vi "Init images and labels.vi"(8 "error in (no error)":errorcluster, 9 "JSON Read":T1, 10 "References":T3, 11 "ControlsIndicators":T5) -> (0 "error out":errorcluster)   [LabVIEW 2019, in "ZenGage v3.0 UI.lvclass"]
uses:
  ZenGage v3.0 UI.lvclass
  Type Definitions/Controls and Indicators/Controls and Indicators Cluster.ctl
  Type Definitions/Controls and Indicators/EDL control references.ctl
  Type Definitions/Controls and Indicators/Select a part (combobox).ctl
  Type Definitions/Controls and Indicators/Diagnostics control referencs.ctl
  Type Definitions/Controls and Indicators/Inspection control references.ctl
  Type Definitions/Controls and Indicators/General_Control references.ctl
  Type Definitions/JSON Read/UI JSON read cluster.ctl
  Type Definitions/General/JSONRead.ctl
  Type Definitions/General/Master sample references.ctl
panel:
  out "TL":string
  out "Trigger Diagnostics (TL)":T4(plugin-control)
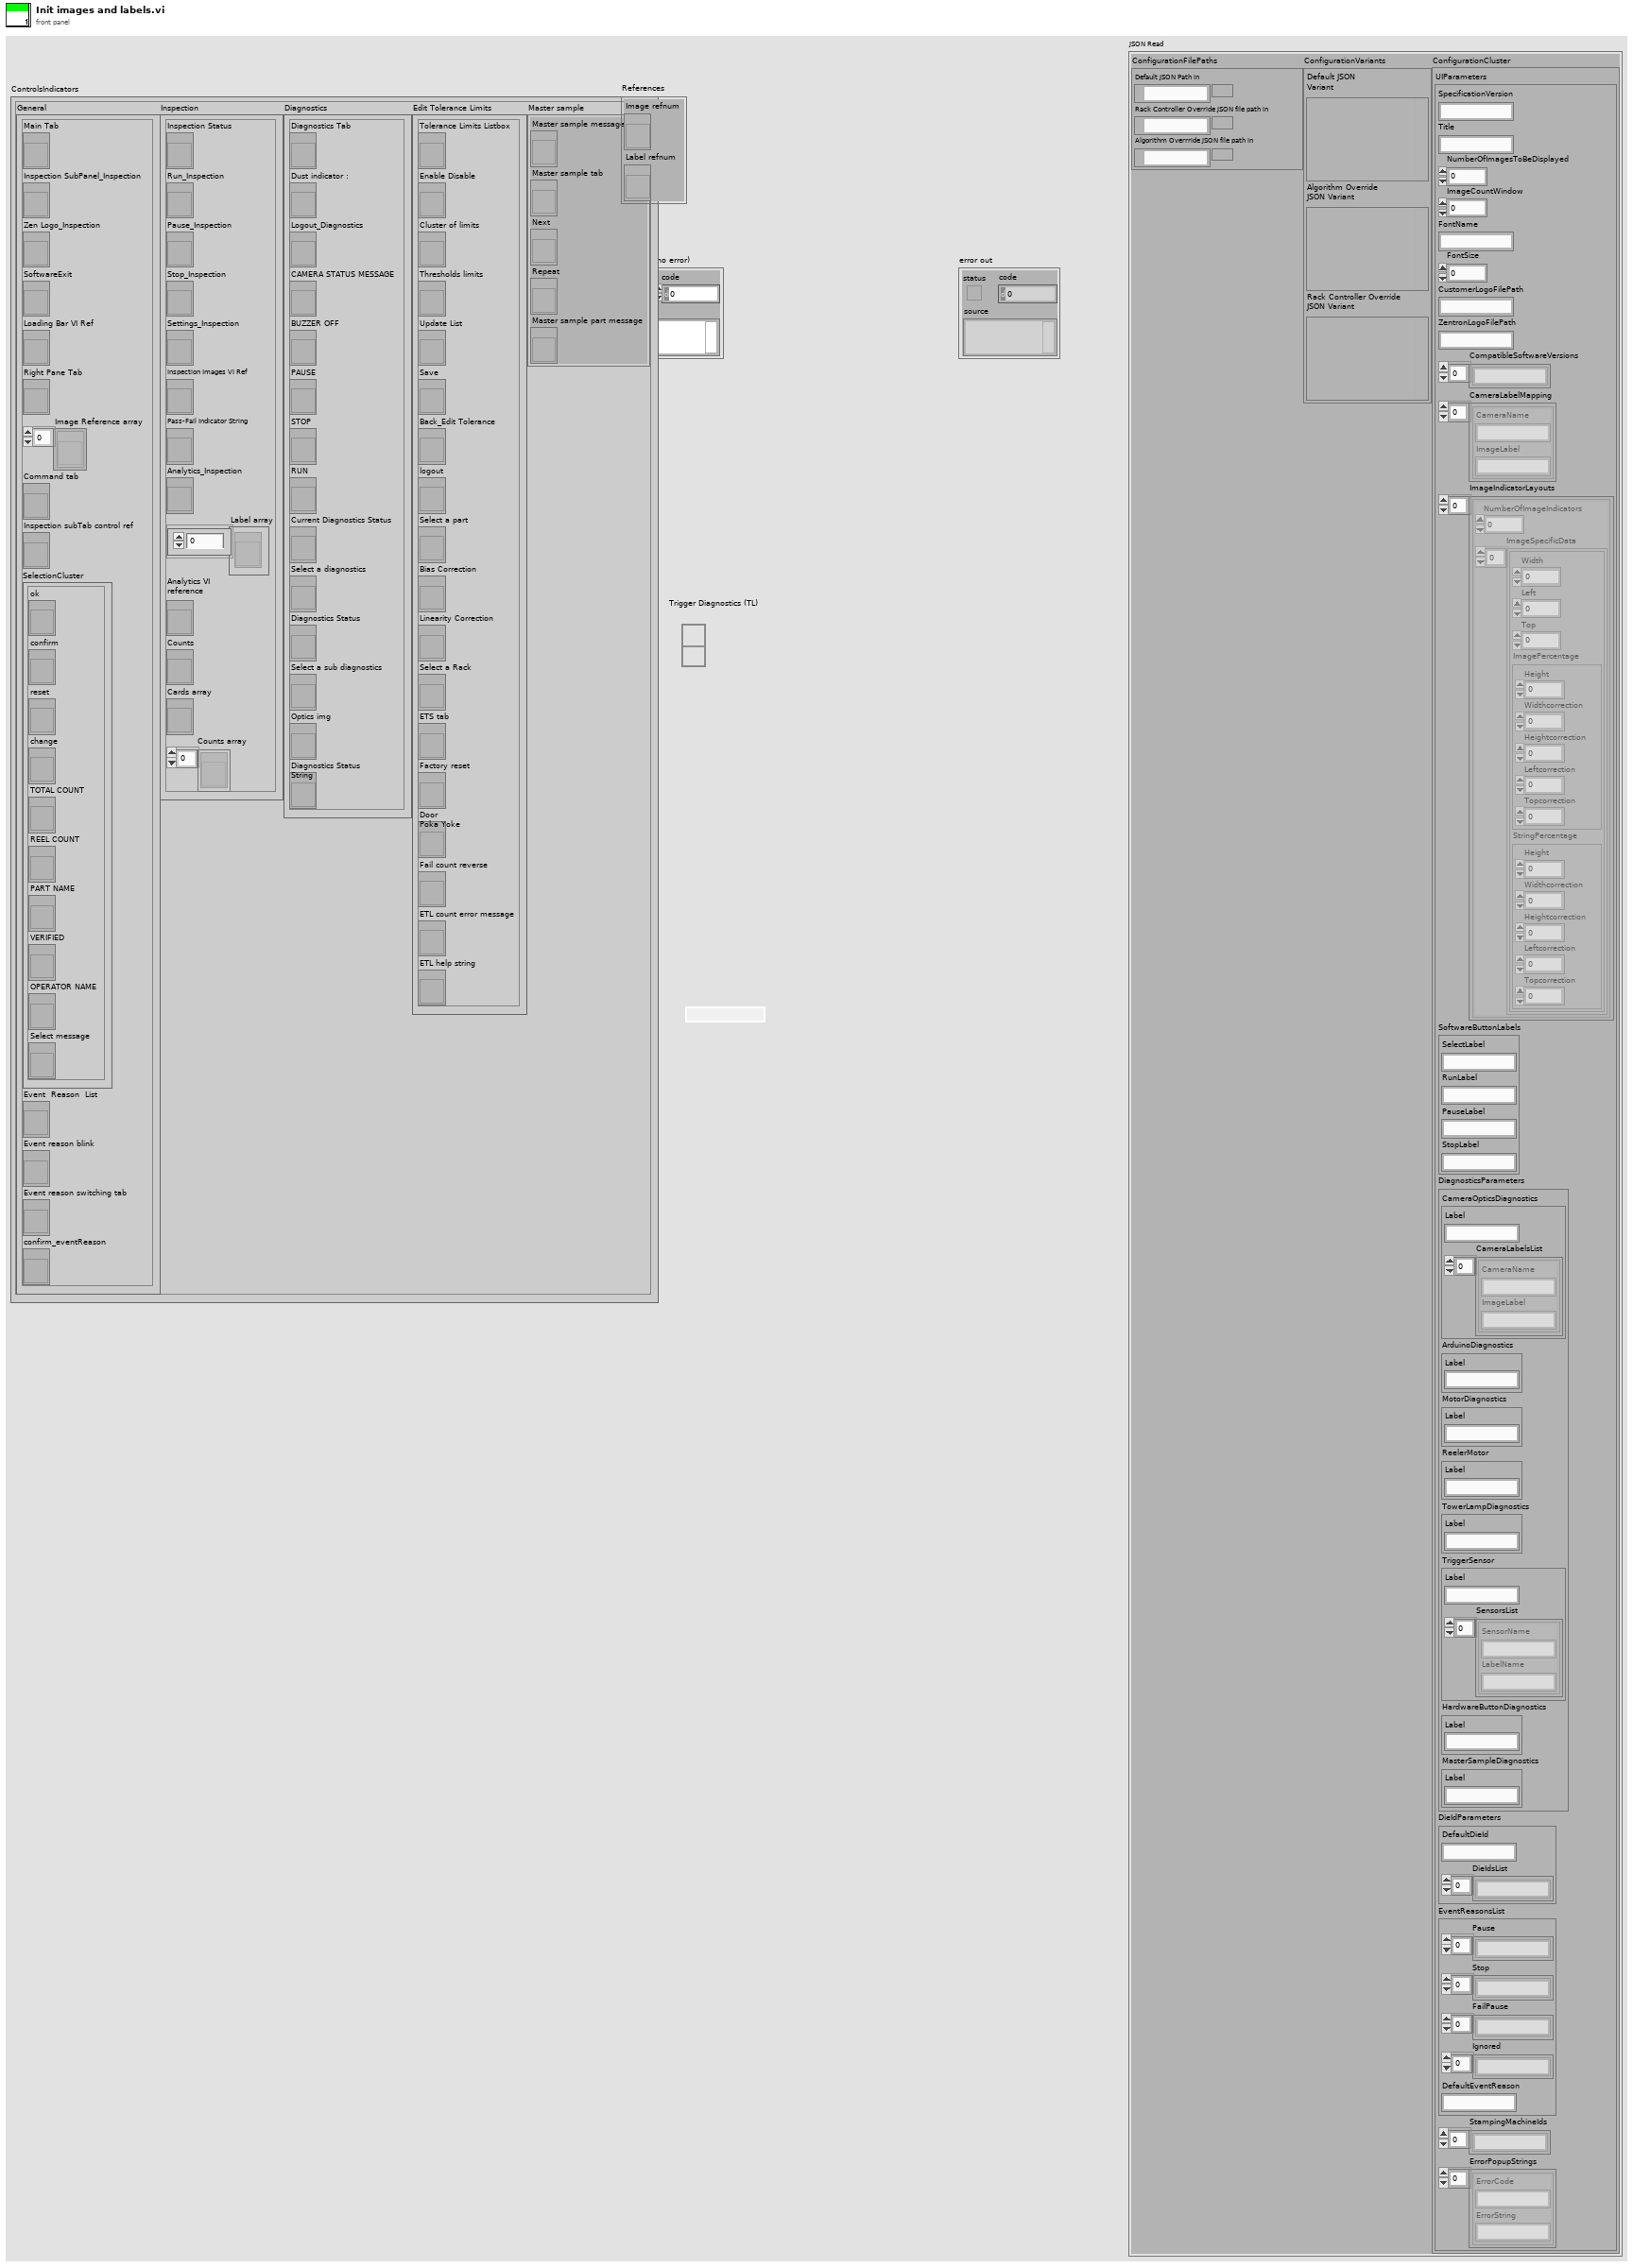
[diagram p1: front panel]
types:
  T1 = typedef "ZenGage v3.0 UI.lvclass/JSONRead.ctl" = cluster{"ConfigurationFilePaths":cluster{"Default JSON Path in":path, "Rack Controller Override JSON file path in":path, "Algorithm Overrride JSON file path in ":path}, "ConfigurationVariants":cluster{"Default JSON \nVariant":variant, "Algorithm Override\nJSON Variant":variant, "Rack Controller Override\nJSON Variant":variant}, "ConfigurationCluster":T2}
  T2 = typedef "ZenGage v3.0 UI.lvclass/UI JSON read cluster.ctl" = cluster{"UIParameters":cluster{"SpecificationVersion":string, "Title":string, "NumberOfImagesToBeDisplayed":dbl, "ImageCountWindow":dbl, "FontName":string, "FontSize":dbl, "CustomerLogoFilePath":string, "ZentronLogoFilePath":string, "CompatibleSoftwareVersions":string[], "CameraLabelMapping":cluster{"CameraName":string, "ImageLabel":string}[], "ImageIndicatorLayouts":cluster{"NumberOfImageIndicators":dbl, "ImageSpecificData":cluster{"Width":dbl, "Left":dbl, "Top":dbl, "ImagePercentage":cluster{"Height":dbl, "Widthcorrection":i64, "Heightcorrection":i64, "Leftcorrection":dbl, "Topcorrection":dbl}, "StringPercentage":cluster{"Height":dbl, "Widthcorrection":i64, "Heightcorrection":dbl, "Leftcorrection":dbl, "Topcorrection":dbl}}[]}[], "SoftwareButtonLabels":cluster{"SelectLabel":string, "RunLabel":string, "PauseLabel":string, "StopLabel":string}, "DiagnosticsParameters":cluster{"CameraOpticsDiagnostics":cluster{"Label":string, "CameraLabelsList":cluster{"CameraName":string, "ImageLabel":string}[]}, "ArduinoDiagnostics":cluster{"Label":string}, "MotorDiagnostics":cluster{"Label":string}, "ReelerMotor":cluster{"Label":string}, "TowerLampDiagnostics":cluster{"Label":string}, "TriggerSensor":cluster{"Label":string, "SensorsList":cluster{"SensorName":string, "LabelName":string}[]}, "HardwareButtonDiagnostics":cluster{"Label":string}, "MasterSampleDiagnostics":cluster{"Label":string}}, "DieIdParameters":cluster{"DefaultDieId":string, "DieIdsList":string[]}, "EventReasonsList":cluster{"Pause":string[], "Stop":string[], "FailPause":string[], "Ignored":string[], "DefaultEventReason":string}, "StampingMachineIds":string[], "ErrorPopupStrings":cluster{"ErrorCode":string, "ErrorString":string}[]}}
  T3 = cluster{"Image refnum":refnum<vi>, "Label refnum":refnum<vi>}
  T4 = typedef "IMAQ Image.ctl" = refnum<image>
  T5 = typedef "ZenGage v3.0 UI.lvclass/Controls and Indicators Cluster.ctl" = cluster{"General":T6, "Inspection":T7, "Diagnostics":T8, "Edit Tolerance Limits":T9, "Master sample":T10}
  T6 = typedef "ZenGage v3.0 UI.lvclass/General_Control references.ctl" = cluster{"Main Tab":refnum<vi>, "Inspection SubPanel_Inspection":refnum<vi>, "Zen Logo_Inspection":refnum<vi>, "SoftwareExit":refnum<vi>, "Loading Bar VI Ref":refnum<vi>, "Right Pane Tab":refnum<vi>, "Image Reference array":refnum<vi>[], "Command tab":refnum<vi>, "Inspection subTab control ref":refnum<vi>, "SelectionCluster":cluster{"ok":refnum<vi>, "confirm":refnum<vi>, "reset":refnum<vi>, "change":refnum<vi>, "TOTAL COUNT":refnum<vi>, "REEL COUNT":refnum<vi>, "PART NAME":refnum<vi>, "VERIFIED":refnum<vi>, "OPERATOR NAME":refnum<vi>, "Select message":refnum<vi>}, "Event  Reason  List":refnum<vi>, "Event reason blink":refnum<vi>, "Event reason switching tab":refnum<vi>, "confirm_eventReason":refnum<vi>}
  T7 = typedef "ZenGage v3.0 UI.lvclass/Inspection control references.ctl" = cluster{"Inspection Status":refnum<vi>, "Run_Inspection":refnum<vi>, "Pause_Inspection":refnum<vi>, "Stop_Inspection":refnum<vi>, "Settings_Inspection":refnum<vi>, "Inspection Images VI Ref":refnum<vi>, "Pass-Fail Indicator String":refnum<vi>, "Analytics_Inspection":refnum<vi>, "Label array":refnum<vi>[], "Analytics VI\nreference":refnum<vi>, "Counts":refnum<vi>, "Cards array":refnum<vi>, "Counts array":refnum<vi>[]}
  T8 = typedef "ZenGage v3.0 UI.lvclass/Diagnostics control referencs.ctl" = cluster{"Diagnostics Tab":refnum<vi>, "Dust indicator :":refnum<vi>, "Logout_Diagnostics":refnum<vi>, "CAMERA STATUS MESSAGE":refnum<vi>, "BUZZER OFF":refnum<vi>, "PAUSE":refnum<vi>, "STOP":refnum<vi>, "RUN":refnum<vi>, "Current Diagnostics Status":refnum<vi>, "Select a diagnostics":refnum<vi>, "Diagnostics Status":refnum<vi>, "Select a sub diagnostics":refnum<vi>, "Optics img":refnum<vi>, "Diagnostics Status\nString":refnum<vi>}
  T9 = typedef "ZenGage v3.0 UI.lvclass/EDL control references.ctl" = cluster{"Tolerance Limits Listbox":refnum<vi>, "Enable Disable":refnum<vi>, "Cluster of limits":refnum<vi>, "Thresholds limits":refnum<vi>, "Update List":refnum<vi>, "Save":refnum<vi>, "Back_Edit Tolerance":refnum<vi>, "logout":refnum<vi>, "Select a part":refnum<vi>, "Bias Correction":refnum<vi>, "Linearity Correction":refnum<vi>, "Select a Rack":refnum<vi>, "ETS tab":refnum<vi>, "Factory reset":refnum<vi>, "Door\nPoka Yoke":refnum<vi>, "Fail count reverse":refnum<vi>, "ETL count error message":refnum<vi>, "ETL help string":refnum<vi>}
  T10 = typedef "Master sample references.ctl" = cluster{"Master sample message":refnum<vi>, "Master sample tab":refnum<vi>, "Next":refnum<vi>, "Repeat":refnum<vi>, "Master sample part message":refnum<vi>}
  T11 = cluster{"Image label ref array":refnum<vi>[], "Image ref array":refnum<vi>[], "Rack 1 Tbl Refnum":refnum<vi>, "Tab control":refnum<vi>, "Rack 2 Tbl Refnum":refnum<vi>, "Image label ref array 2":refnum<vi>[], "Diagnostics tab ref":refnum<vi>}
  T12 = cluster{"NumberOfImageIndicators":dbl, "ImageSpecificData":cluster{"Width":dbl, "Left":dbl, "Top":dbl, "ImagePercentage":cluster{"Height":dbl, "Widthcorrection":i64, "Heightcorrection":i64, "Leftcorrection":dbl, "Topcorrection":dbl}, "StringPercentage":cluster{"Height":dbl, "Widthcorrection":i64, "Heightcorrection":dbl, "Leftcorrection":dbl, "Topcorrection":dbl}}[]}[]
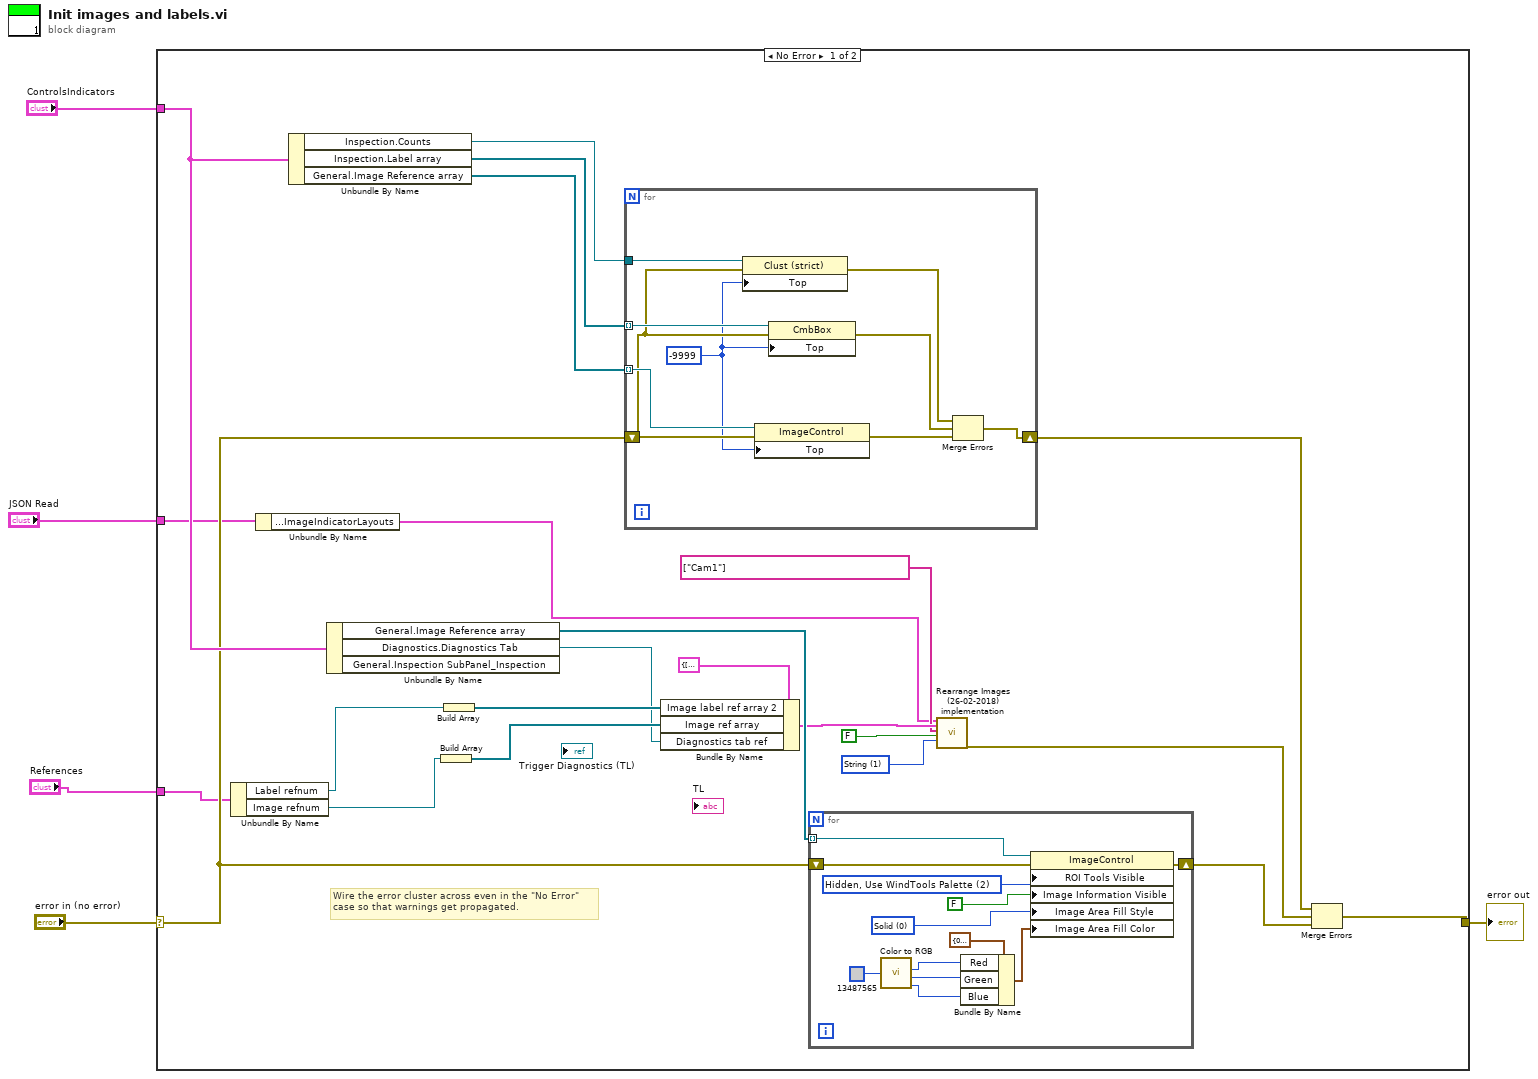
[diagram p0: block diagram]
diagram:
  n1 = case shown="No Error" "error in (no error)" {
    selector: "error in (no error)" -> [w17 w50]
    tunnel: [w26 w50] -> w4
    tunnel: "ControlsIndicators" -> [w18 _]
    tunnel: "References" -> [w12 _]
    tunnel: "JSON Read" -> [w8 _]
    frame No Error {
      w19 = u16 1 items=["Combo", "String"] ("Type of label")
      # "Wire the error cluster across even in the \"No Error\"\ncase so that warnings get propagated."
      n2 = Unbundle By Name(w12) -> ("Label refnum"=w11:refnum<vi>, "Image refnum"=w10:refnum<vi>)
      n3 = Unbundle By Name(w8) -> ("ConfigurationCluster.UIParameters.ImageIndicatorLayouts"=w7:T12)
      n4 = Unbundle By Name(w18) -> ("Inspection.Counts"=w6:refnum<vi>, "Inspection.Label array"=w28:refnum<vi>[], "General.Image Reference array"=w27:refnum<vi>[])
      n5 = Unbundle By Name(w18) -> ("General.Image Reference array"=w25:refnum<vi>[], "Diagnostics.Diagnostics Tab"=w21:refnum<vi>)  [unwired: 1 out]
      n6 = Build Array(w10) -> (w24:refnum<vi>[])
      n7 = Build Array(w11) -> (w23:refnum<vi>[])
      n8 = for {
        tunnel: w28 -> [w49] mode=indexing
        tunnel: w27 -> [w48] mode=indexing
        shift-right: [w45] -> w15
        shift-left: w17 -> [w43]
        tunnel: w6 -> [w44]
        w42 = -9999 ("Position:Top")
        n9 = property class="Clust (strict)"(reference=w44, error in=w43, "Top"=w42) -> (error out=w41:errorcluster)  [unwired: 1 out]
        n10 = property class="ImageControl"(reference=w48, error in=w43, "Top"=w42) -> (error out=w47:errorcluster)  [unwired: 1 out]
        n11 = property class="CmbBox"(reference=w49, error in=w43, "Top"=w42) -> (error out=w46:errorcluster)  [unwired: 1 out]
        n12 = Merge Errors(w41, w46, w47) -> (w45:errorcluster)
      }
      n13 = Bundle By Name(cluster=T11 {"Image label ref array"=[], "Image ref array"=[refnum], "Rack 1 Tbl Refnum"=refnum, "Tab control"=refnum, "Rack 2 Tbl Refnum"=refnum, "Image label ref array 2"=[], "Diagnostics tab ref"=refnum} ("References"), "Image label ref array 2"=w23, "Image ref array"=w24, "Diagnostics tab ref"=w21) -> (w13:T11)
      n14 = for {
        tunnel: w25 -> [w40] mode=indexing
        shift-right: [w37] -> w16
        shift-left: w17 -> [w38]
        w35 = u32 0 items=["Default"=3, "Solid"=0, "Hatch"=2] ("Image Area:Background:Fill Style")
        w39 = u32 2 items=["Visible", "Hidden", "Hidden, Use WindTools Palette"] ("ROI Tools Visible")
        n15 = call <vilib>:"Color to RGB.vi"("Color"=u32 13487565) -> ("R"=w32:u8, "G"=w31:u8, "B"=w30:u8)  [unwired: 1 out]
        n16 = Bundle By Name(cluster=cluster{"Red":u8, "Green":u8, "Blue":u8} {"Red"=0, "Green"=0, "Blue"=0} ("Image Area:Background:Fill Color"), "Red"=w32, "Green"=w31, "Blue"=w30) -> (w29:cluster{"Red":u8, "Green":u8, "Blue":u8})
        n17 = property class="ImageControl"(reference=w40, error in=w38, "ROI Tools Visible"=w39, "Image Information Visible"=FALSE, "Image Area Fill Style"=w35, "Image Area Fill Color"=w29) -> (error out=w37:errorcluster)  [unwired: 1 out]
      }
      n18 = call "Rearrange Images (26-02-2018) implementation.vi"("Image indicator layouts 2"=w7, "References"=w13, "Camera names"=string[] ["Cam1"], "Update\nTables"=FALSE ("Update\nTables"), "Type of label"=w19) -> ("error out"=w14:errorcluster)  [unwired: 14 in]
      n19 = Merge Errors(w15, w14, w16) -> (w26:errorcluster)
    }
    frame Error {
    }
  }
  "error out" <- w4
